vi "Untitled 1.vi"() -> ()   [LabVIEW 2022 SP3]
panel:
  out "Pedstrian green":bool
  out "Pedstrian red":bool
  in  "stop":bool
  in  "Push":bool
  out "Green":bool
  out "Yellow":bool
  out "Red":bool
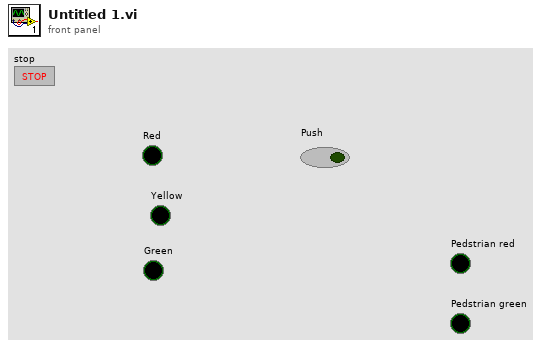
[diagram p1: front panel]
types:
  T1 = enum16{"Initial", "Wait Inputs", "Push", "State 4", "State 5"}
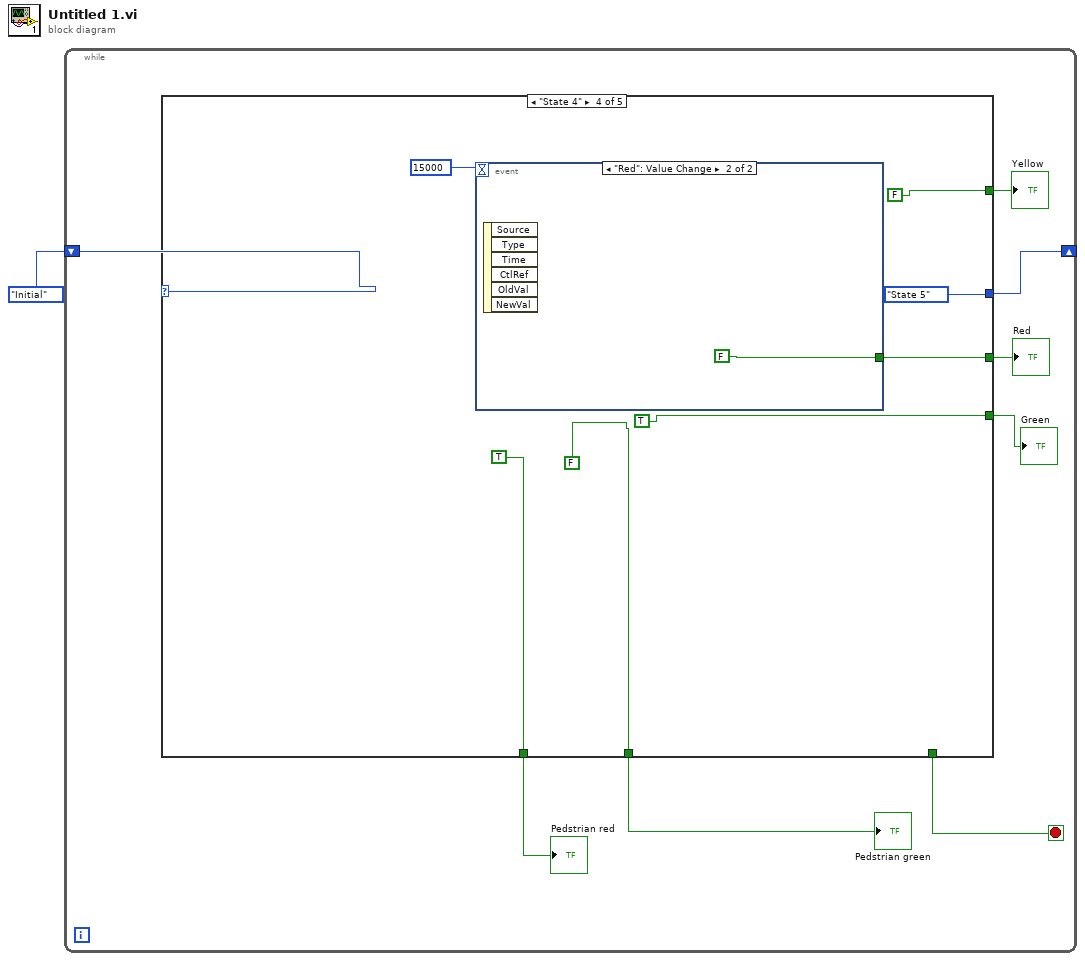
[diagram p0: block diagram]
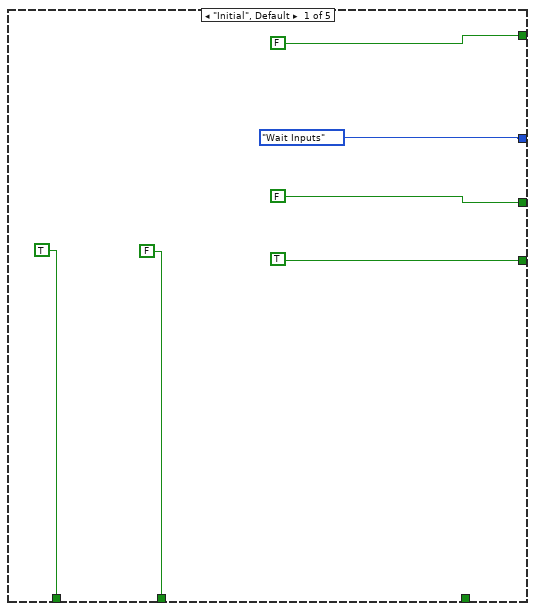
[diagram p2: hidden frame]
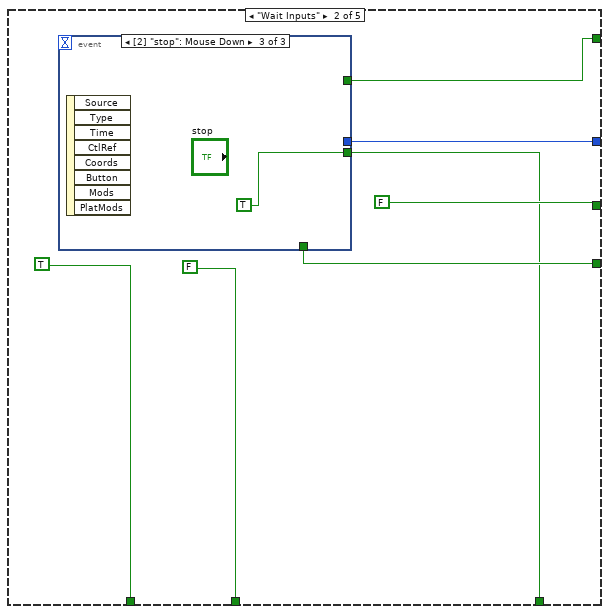
[diagram p3: hidden frame]
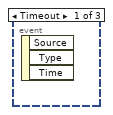
[diagram p4: hidden frame]
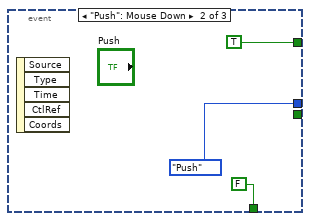
[diagram p5: hidden frame]
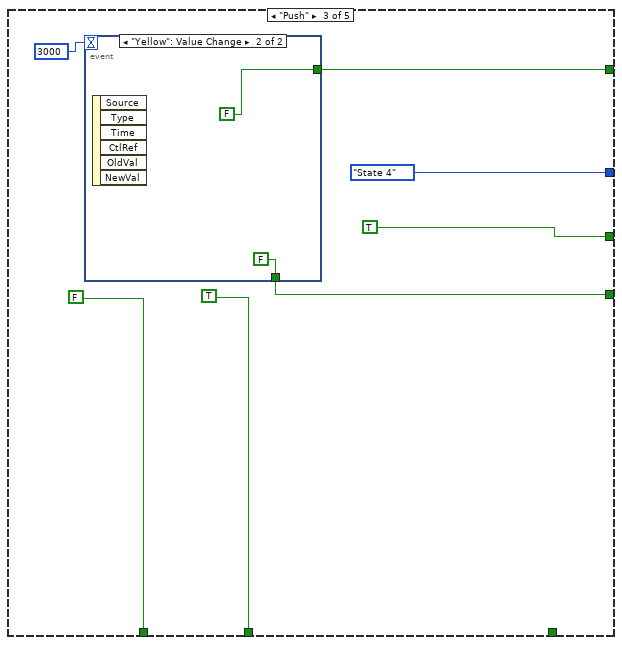
[diagram p6: hidden frame]
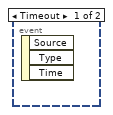
[diagram p7: hidden frame]
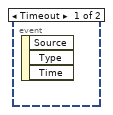
[diagram p8: hidden frame]
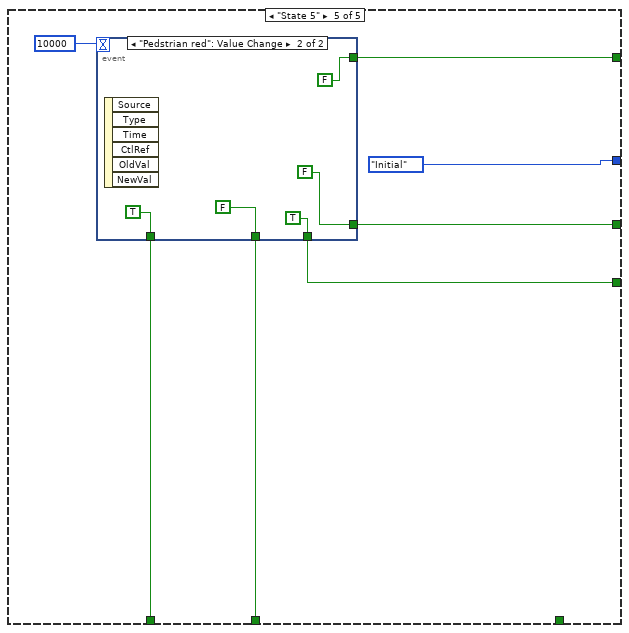
[diagram p9: hidden frame]
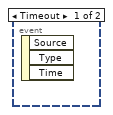
[diagram p10: hidden frame]
diagram:
  n1 = while {
    shift-right: [w8] -> _
    shift-left: T1."Initial" -> [w9]
    stop <- w2 stop-if-true
    n2 = case shown="\"State 4\"" w9 {
      tunnel: [T1."Wait Inputs" w22 T1."State 4" T1."State 5" T1."Initial"] -> w8
      tunnel: [FALSE w21 w33 FALSE w46] -> w7
      tunnel: [FALSE FALSE TRUE w42 w45] -> w6
      tunnel: [TRUE w19 w31 TRUE w44] -> w5
      tunnel: [TRUE TRUE FALSE TRUE w48] -> w4
      tunnel: [FALSE FALSE TRUE FALSE w47] -> w3
      tunnel: [_ w16 _ _ _] -> w2
      frame "Initial", Default {
      }
      frame "Wait Inputs" {
        n3 = event shown="[2] \"stop\": Mouse Down" {
          selector: _ -> [_ _ _]
          dyn-events: _ -> [_ _ _]
          timeout: _ -> [_ _ _]
          tunnel: [_ T1."Push" _] -> w22
          tunnel: [_ TRUE _] -> w21
          tunnel: [_ FALSE _] -> w19
          tunnel: [_ _ TRUE] -> w16
          event Timeout {
            n4 = event-data() -> ()  [unwired: 1 in, 3 out]
          }
          event "Push": Mouse Down {
            n5 = event-data() -> ()  [unwired: 1 in, 5 out]
          }
          event "stop": Mouse Down {
            n6 = event-data() -> ()  [unwired: 1 in, 8 out]
          }
        }
      }
      frame "Push" {
        n7 = event shown="[1] \"Yellow\": Value Change" {
          selector: _ -> [_ _]
          dyn-events: _ -> [_ _]
          timeout: 3000 -> [_ _]
          tunnel: [_ FALSE] -> w33
          tunnel: [_ FALSE] -> w31
          event Timeout {
            n8 = event-data() -> ()  [unwired: 1 in, 3 out]
          }
          event "Yellow": Value Change {
            n9 = event-data() -> ()  [unwired: 1 in, 6 out]
          }
        }
      }
      frame "State 4" {
        n10 = event shown="[1] \"Red\": Value Change" {
          selector: _ -> [_ _]
          dyn-events: _ -> [_ _]
          timeout: 15000 -> [_ _]
          tunnel: [_ FALSE] -> w42
          event Timeout {
            n11 = event-data() -> ()  [unwired: 1 in, 3 out]
          }
          event "Red": Value Change {
            n12 = event-data() -> ()  [unwired: 1 in, 6 out]
          }
        }
      }
      frame "State 5" {
        n13 = event shown="[1] \"Pedstrian red\": Value Change" {
          selector: _ -> [_ _]
          dyn-events: _ -> [_ _]
          timeout: 10000 -> [_ _]
          tunnel: [_ TRUE] -> w48
          tunnel: [_ FALSE] -> w47
          tunnel: [_ FALSE] -> w46
          tunnel: [_ FALSE] -> w45
          tunnel: [_ TRUE] -> w44
          event Timeout {
            n14 = event-data() -> ()  [unwired: 1 in, 3 out]
          }
          event "Pedstrian red": Value Change {
            n15 = event-data() -> ()  [unwired: 1 in, 6 out]
          }
        }
      }
    }
    "Yellow" <- w7
    "Red" <- w6
    "Green" <- w5
    "Pedstrian green" <- w3
    "Pedstrian red" <- w4
  }
